vi "FGV_REWORK_connection_indicators.vi"(4 "PLC_connections_indicator_global":refnum<vi>, 6 "SQL_connections_indicator_global":refnum<vi>, 7 "options":T1, 8 "error_in":errorcluster, 11 "status":bool) -> (0 "error_out":errorcluster)   [LabVIEW 2019]
uses:
  FGV_REWORK_connection_indicators.ctl
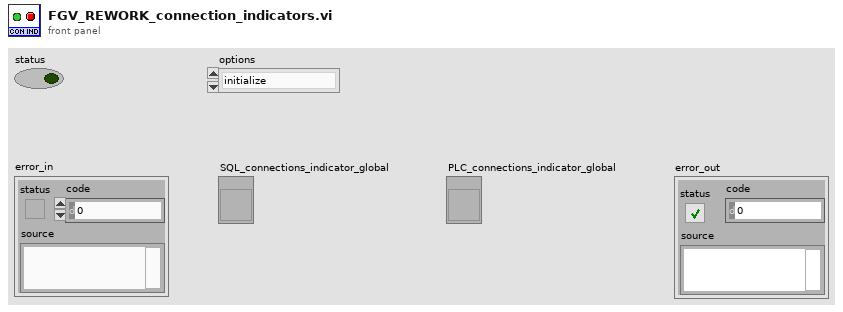
[diagram p1: front panel]
types:
  T1 = typedef "FGV_REWORK_connection_indicators.ctl" = enum16{"initialize", "SQL_conn_ind_update", "PLC_conn_ind_update"}
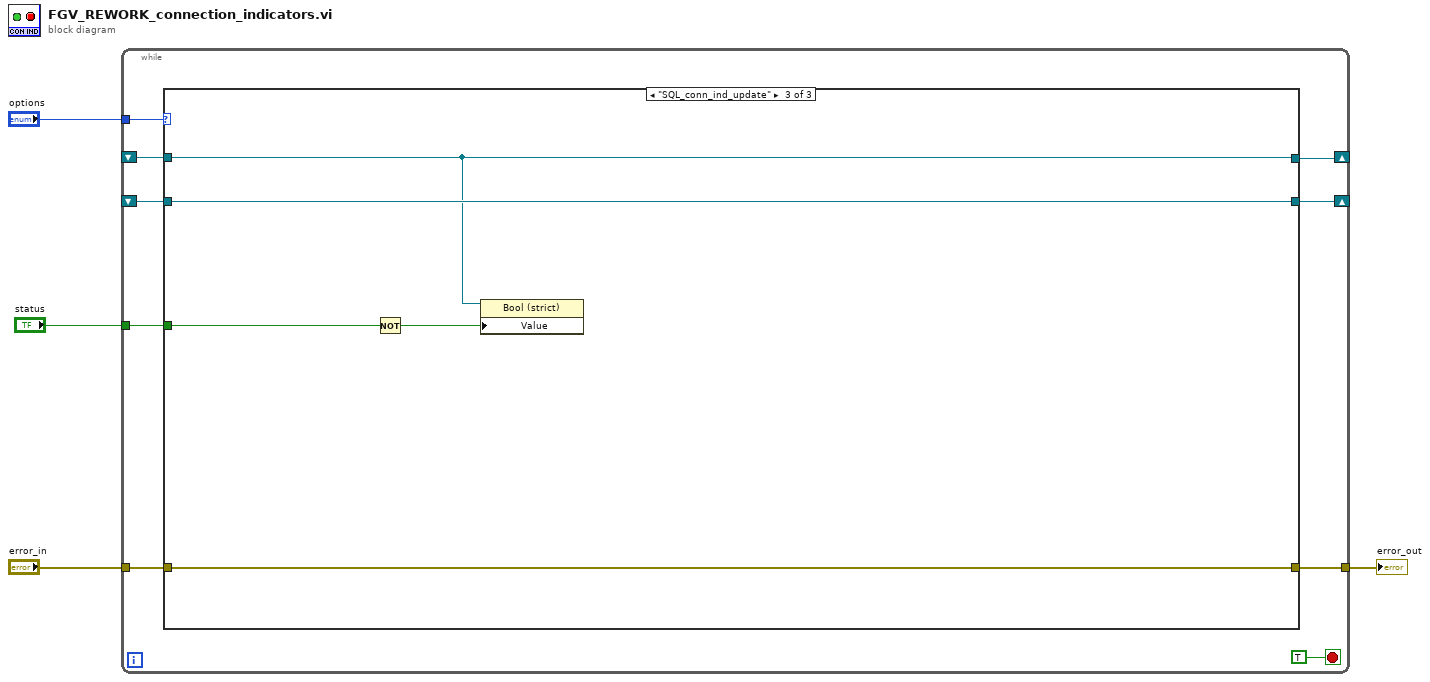
[diagram p0: block diagram]
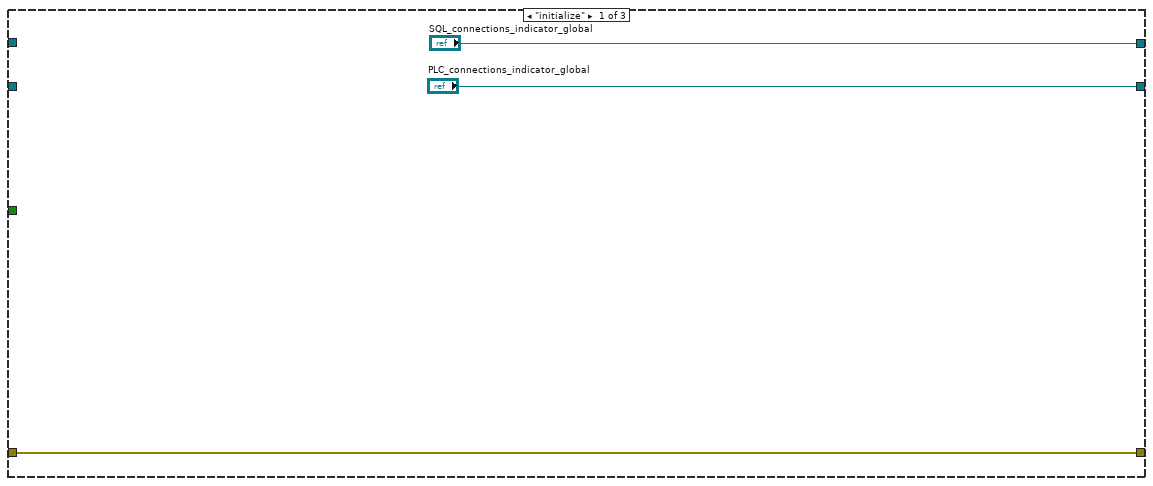
[diagram p2: hidden frame]
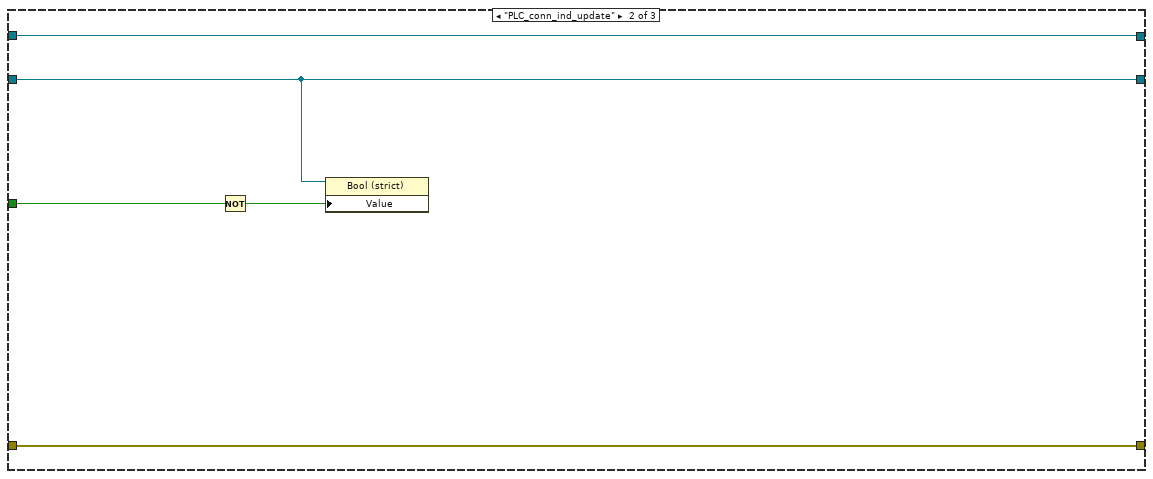
[diagram p3: hidden frame]
diagram:
  n1 = while {
    tunnel: "options" -> [w12]
    tunnel: [w11] -> w4
    tunnel: "error_in" -> [w10]
    shift-right: [w9] -> _
    shift-left: _ -> [w7]
    shift-right: [w8] -> _
    shift-left: _ -> [w6]
    tunnel: "status" -> [w5]
    stop <- TRUE stop-if-true
    n2 = case shown="\"SQL_conn_ind_update\"" w12 {
      tunnel: [w16 w21 w26] -> w11
      tunnel: w10 -> [w16 w21 w26]
      tunnel: ["SQL_connections_indicator_global" w20 w23] -> w9
      tunnel: ["PLC_connections_indicator_global" w19 w25] -> w8
      tunnel: w7 -> [_ w20 w23]
      tunnel: w6 -> [_ w19 w25]
      tunnel: w5 -> [_ w17 w22]
      frame "initialize" {
      }
      frame "PLC_conn_ind_update" {
        n3 = Not(x=w17) -> (.not. x?=w18:bool)
        n4 = property class="Bool (strict)"(reference=w19, "Value"=w18) -> ()  [unwired: 1 in, 2 out]
      }
      frame "SQL_conn_ind_update" {
        n5 = Not(x=w22) -> (.not. x?=w24:bool)
        n6 = property class="Bool (strict)"(reference=w23, "Value"=w24) -> ()  [unwired: 1 in, 2 out]
      }
    }
  }
  "error_out" <- w4
